vi "DriveShifter.vi"(8 "error in (no error)":errorcluster, 10 "HighGear?":bool, 11 "Drive in":refnum<class "Drive.lvclass">) -> (0 "error out":errorcluster, 3 "Drive out":refnum<class "Drive.lvclass">)   [LabVIEW 2018, in "Drive.lvlib" / "Drive.lvclass"]
doc: "This VI switches the pneumatic piston from HIGH to LOW depending on the boolean that arrives. If the boolean does not change, and the switching time has elapsed, then it will keep the solenid off."
uses:
  Drive.lvclass
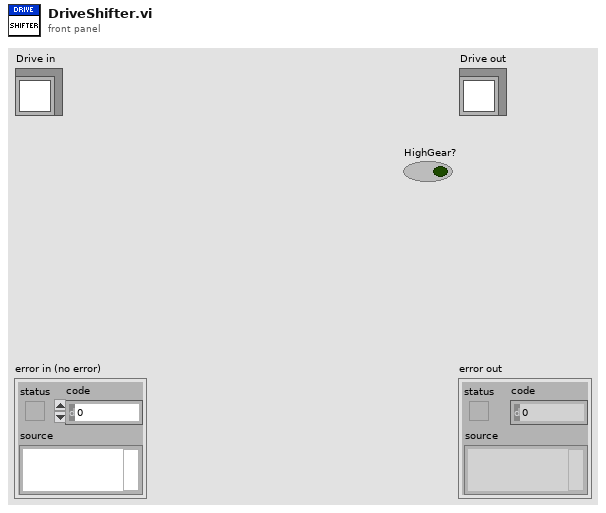
[diagram p1: front panel]
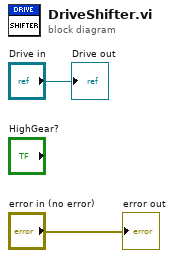
[diagram p0: block diagram]
diagram:
  "error out" <- "error in (no error)"
  "Drive out" <- "Drive in"
